vi "Init Serial Port.vi"(8 "error in (no error)":errorcluster, 9 "Input\nbuffer size":u32=4096, 10 "baud rate":u32=9600, 11 "VISA Refnum in":refnum<visa-resource-name>) -> (0 "error out":errorcluster, 3 "VISA Refnum out":refnum<visa-resource-name>)   [LabVIEW 2013]
doc: "opens a serial port (on the RIO or a standard computer) and sets up the buffers so they actually work.\n-Jason"
uses:
  <vilib>/Instr/_visa.llb/VISA Configure Serial Port (Instr).vi
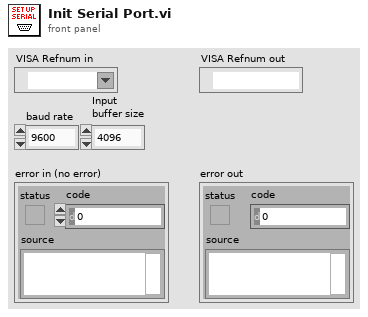
[diagram p1: front panel]
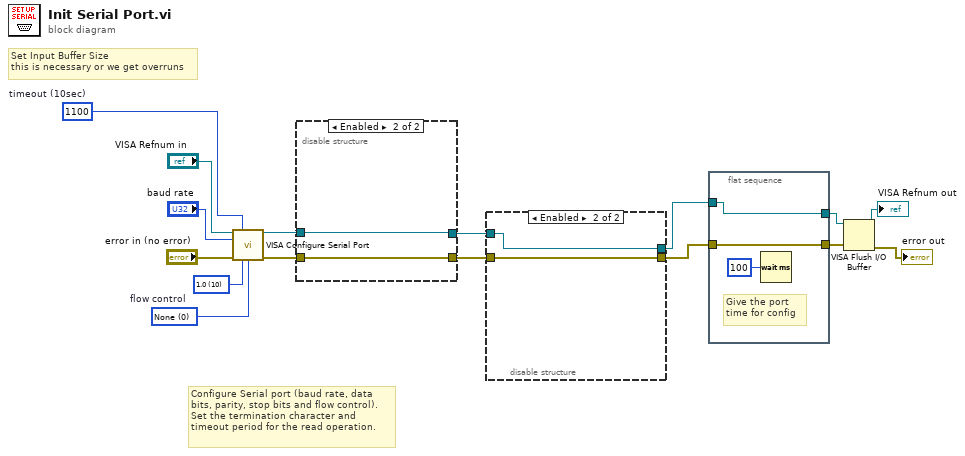
[diagram p0: block diagram]
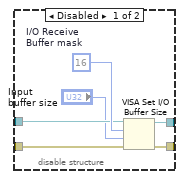
[diagram p2: hidden frame]
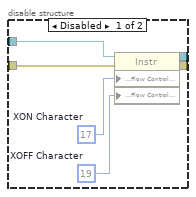
[diagram p3: hidden frame]
diagram:
  w8 = u16 10 items=["1.0"=10, "1.5"=15, "2.0"=20] ("stop bits (10: 1 bit)")
  w14 = u32 1100  # timeout (10sec)
  w10 = u16 0 items=["None"=0, "XON/XOFF"=1, "RTS/CTS"=2, "DTR/DSR"=4]  # flow control
  # "Set Input Buffer Size\nthis is necessary or we get overruns"
  # "Configure Serial port (baud rate, data\nbits, parity, stop bits and flow control).\nSet the termination character and\ntimeout period for the read operation."
  n1 = call-poly "VISA Configure Serial Port"("VISA resource name"="VISA Refnum in", "timeout (10sec)"=w14, "baud rate (9600)"="baud rate", "error in (no error)"="error in (no error)", "stop bits (10: 1 bit)"=w8, "flow control (0:none)"=w10) -> ("VISA resource name out"=w12:refnum<visa-resource-name>, "error out"=w13:errorcluster)  [unwired: 8 in]
  n2 = disable-structure shown="Enabled" {
    disable-tunnel: w13 -> [w21 w23]
    disable-tunnel: w12 -> [w20 w24]
    disable-tunnel: [w19 w24] -> w11
    disable-tunnel: [w17 w23] -> w7
    frame Disabled {
      w22 = u16 16  # I/O Receive Buffer mask
      n3 = VISA Set I/O Buffer Size(VISA resource name=w20, mask (16)=w22, size (4096)="Input\nbuffer size", error in (no error)=w21) -> (VISA resource name out=w19:refnum<visa-resource-name>, error out=w17:errorcluster)
    }
    frame Enabled {
    }
  }
  n4 = disable-structure shown="Enabled" {
    disable-tunnel: [w30 w31] -> w5
    disable-tunnel: [w29 w32] -> w6
    disable-tunnel: w11 -> [w25 w32]
    disable-tunnel: w7 -> [w26 w31]
    frame Disabled {
      w28 = u8 19  # XOFF Character
      w27 = u8 17  # XON Character
      n5 = property class="Instr"(reference=w25, error in=w26, "Serial Settings:Flow Control XON Character"=w27, "Serial Settings:Flow Control XOFF Character"=w28) -> (reference out=w29:refnum<visa-resource-name>, error out=w30:errorcluster)
    }
    frame Enabled {
    }
  }
  n6 = flat-sequence {
    tunnel: w6 -> [w34]
    tunnel: [w34] -> w3
    tunnel: w5 -> [w33]
    tunnel: [w33] -> w4
    frame #0 {
      # "Give the port\ntime for config"
      n7 = Wait (ms)(milliseconds to wait=u32 100) -> ()  [unwired: 1 out]
    }
  }
  n8 = VISA Flush I/O Buffer(VISA resource name=w3, error in (no error)=w4) -> (VISA resource name out=→"VISA Refnum out":refnum<visa-resource-name>, error out=→"error out":errorcluster)  [unwired: 1 in]
